vi "RTS Find Sequencial Datasets.vi"(8 "Error In":errorcluster, 11 "File Location":path) -> (0 "Error Out":errorcluster, 2 "Full Data List":path[](array[path]), 3 "Organized File Open List":path[](array[path]))   [LabVIEW 2016]
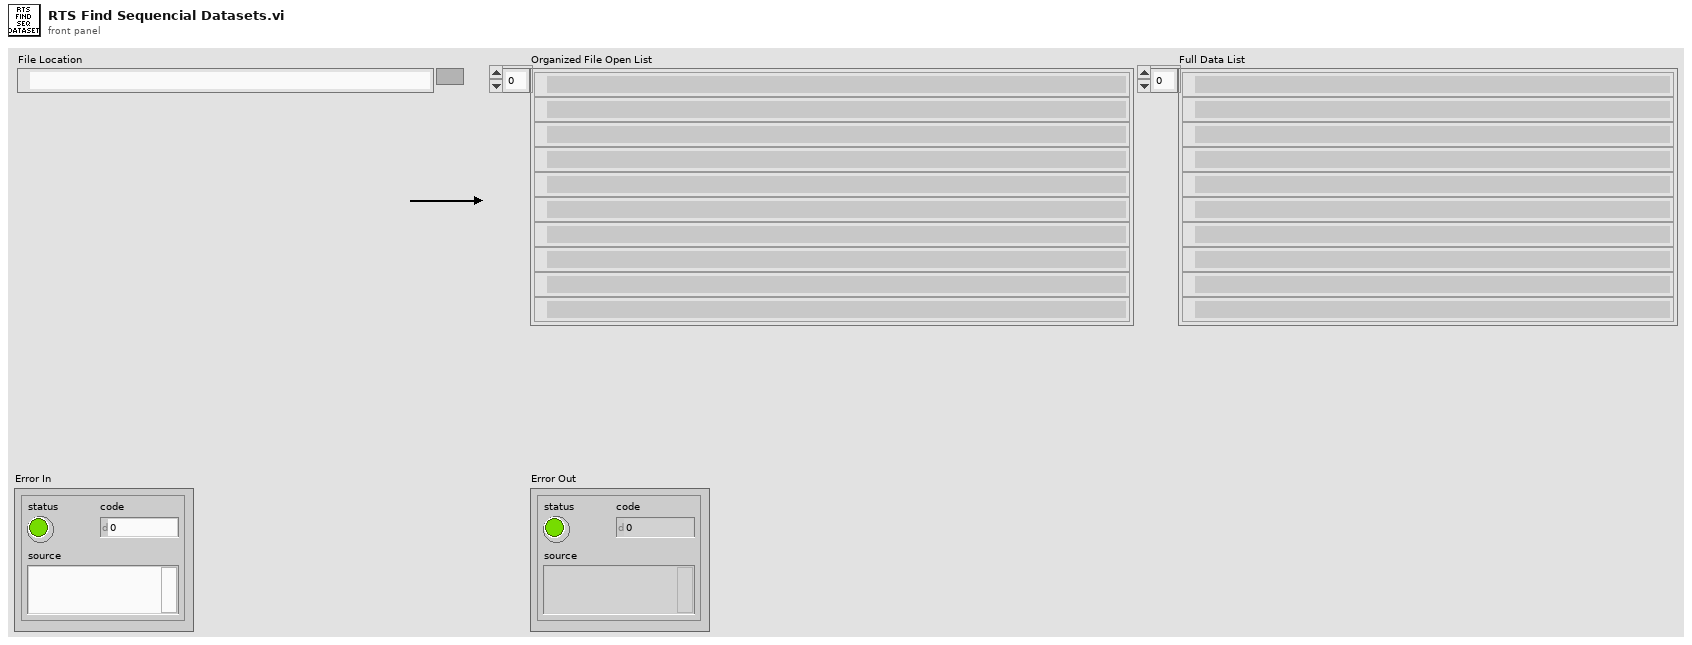
[diagram p1: front panel]
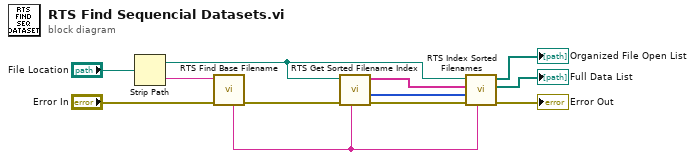
[diagram p0: block diagram]
diagram:
  n1 = Strip Path(path="File Location") -> (stripped path=w10:path, name=w11:string)
  n2 = call "RTS Find Base Filename.vi"("Error In"="Error In", "Input name"=w11) -> ("Error Out"=w9:errorcluster, "Base File Name"=w6:string)  [unwired: 8 in]
  n3 = call "RTS Get Sorted Filename Index.vi"("Base File Name"=w6, "Error In"=w9, "stripped path"=w10) -> ("Error Out"=w7:errorcluster, "Sorted Filename index"=w4:i32[], "filenames"=w5:string[])  [unwired: 6 in]
  n4 = call "RTS Index Sorted Filenames.vi"("Base File Name"=w6, "Error In"=w7, "Sorted Filename index"=w4, "filenames"=w5, "stripped path"=w10) -> ("Error Out"=→"Error Out":errorcluster, "Full Data List"=→"Full Data List":path[], "Organized File Open List"=→"Organized File Open List":path[])  [unwired: 4 in]
